vi "FormatStringArray.vi"(0 "strings":string[](array[string]), 1 "string encoding":enum16{"None", "Base64"}(ring)=enum."Base64") -> (2 "value":string)   [LabVIEW 2014, in "PythonConfiguration.lvclass"]
uses:
  PythonConfiguration.lvclass
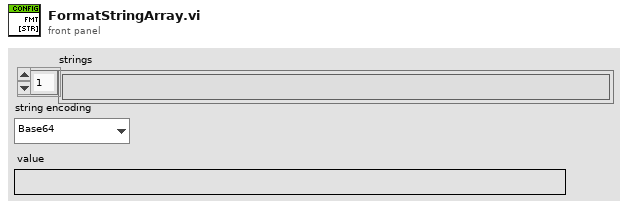
[diagram p1: front panel]
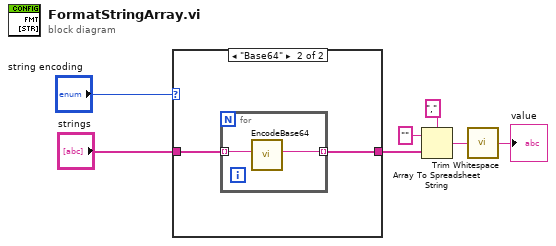
[diagram p0: block diagram]
diagram:
  n1 = case shown="\"Base64\"" "string encoding" {
    tunnel: "strings" -> [w8 w10]
    tunnel: [w8 w9] -> w5
    frame "None" {
    }
    frame "Base64" {
      n2 = for {
        tunnel: w10 -> [w12] mode=indexing
        tunnel: [w11] -> w9 mode=indexing
        n3 = call "EncodeBase64.vi"("string"=w12) -> ("base64 string"=w11:string)  [unwired: 10 in]
      }
    }
  }
  n4 = Array To Spreadsheet String(delimiter (Tab)=",", array=w5, 3:"" ("format string")) -> (spreadsheet string=w2:string)
  n5 = call <vilib>:"Trim Whitespace.vi"("string"=w2) -> ("trimmed string"=→"value":string)  [unwired: 1 in]
